vi "Get Osc Support Samples.vi"(10 "maxnum":i32, 11 "sample":u32[](array[numeric])=[0, 0, 0, 0, 0, 0, 0, 0, 0, 0, 0, 0, 0, 0, 0, 0, 0, 0, 0, 0]) -> (2 "function return":i32, 3 "sample out":u32[](array[numeric]))   [LabVIEW 2021, in "vmmso.lvlib"]
doc: "DLL_API int WINAPI GetOscSupportSamples(unsigned int* sample, int maxnum);"
uses:
  vmmso.lvlib
  vmmso.dll
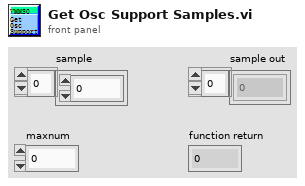
[diagram p1: front panel]
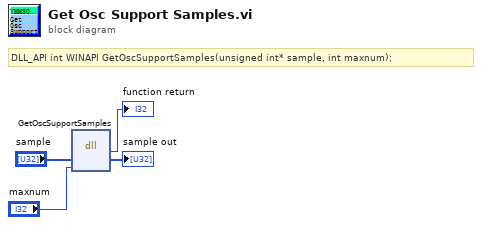
[diagram p0: block diagram]
diagram:
  # "DLL_API int WINAPI GetOscSupportSamples(unsigned int* sample, int maxnum);"
  n1 = dll-call lib="D:/labviewdemo/LabviewDemo 21/vmmso/vmmso.*" fn="GetOscSupportSamples"("sample"="sample", "maxnum"="maxnum") -> (→"function return":i32, "sample"=→"sample out":u32[])  [unwired: 4 in, 2 out]
